vi "ErrorMngmt_Open.vi"() -> (0 "error out":errorcluster, 3 "Queue out":refnum<queue>)   [LabVIEW 2015]
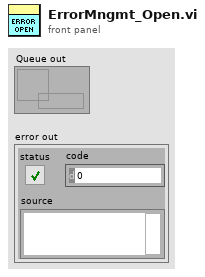
[diagram p1: front panel]
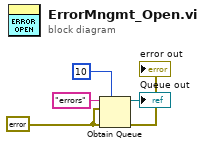
[diagram p0: block diagram]
diagram:
  w3 = errorcluster {"status"=FALSE, "code"=0, "source"=""} ("error constant")
  n1 = Obtain Queue(max queue size (-1, unlimited)=10, name (unnamed)="errors", element data type=w3, error in (no error)=w3) -> (queue out=→"Queue out":refnum<queue>, error out=→"error out":errorcluster)  [unwired: 1 in, 1 out]
